vi "CustomizedDialog.vi"(8 "error in (no error)":errorcluster) -> (0 "error out":errorcluster)   [LabVIEW 2020]
panel:
  in  "OK":bool
  out "Error Message":string
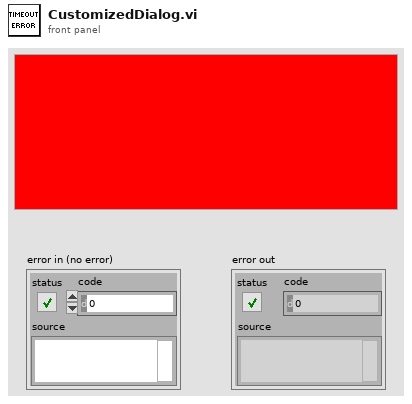
[diagram p1: front panel]
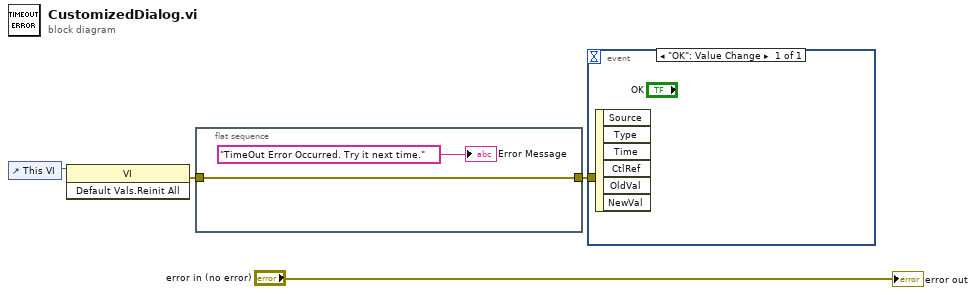
[diagram p0: block diagram]
diagram:
  n1 = control-ref of="This VI"() -> (w3:refnum<vi>)
  n2 = invoke class="VI" method="Default Vals.Reinit All"(reference=w3) -> (error out=w2:errorcluster)  [unwired: 2 in, 2 out]
  n3 = flat-sequence {
    tunnel: w2 -> [w5]
    tunnel: [w5] -> w1
    frame #0 {
      "Error Message" <- "TimeOut Error Occurred. Try it next time." ("Error Message")
    }
  }
  n4 = event shown="[0] \"OK\": Value Change" {
    selector: _ -> [_]
    dyn-events: _ -> [_]
    timeout: _ -> [_]
    tunnel: w1 -> [_]
    event "OK": Value Change {
      n5 = event-data() -> ()  [unwired: 1 in, 6 out]
    }
  }
  "error out" <- "error in (no error)"
